vi "InitTwoStack.vi"(8 "Second":refnum<class "ActionStack.lvclass">, 9 "ActionStack in":refnum<class "ActionStack.lvclass">) -> (1 "Actions":refnum<class "ActionStack.lvclass">[](array[class]))   [LabVIEW 2024, in "ActionStack.lvclass"]
uses:
  ActionStack.lvclass
  ActionStack.lvclass/ActionStack.ctl
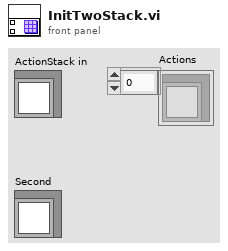
[diagram p1: front panel]
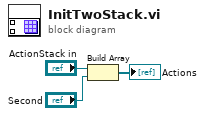
[diagram p0: block diagram]
diagram:
  n1 = Build Array("ActionStack in", "Second") -> (→"Actions":refnum<class "ActionStack.lvclass">[])
